vi "Configure Frequency Sweep.vi"(0 "VISA resource name":refnum<visa-resource-name>, 1 "Stop  Frequency (1000 Hz)":dbl=1000.0, 2 "Sweep Hold Time (0 s)":dbl, 5 "Sweep Spacing (0: Linear)":i32(ring) items=["Linear", "Log"], 7 "Sweep Time (1 s)":dbl=1.0, 9 "Channel (1: 1)":i32(ring)=1 items=["1"=1, "2"=2], 11 "error in (no error)":errorcluster, 12 "Start Frequency (100 Hz)":dbl=100.0, 13 "Sweep Return Time (0 s)":dbl) -> (4 "VISA resource name out":refnum<visa-resource-name>, 15 "error out":errorcluster)   [LabVIEW 2019, in "Agilent 3352X Series.lvlib"]
doc: "Configures for a frequency sweep. In the frequency sweep mode, the function generator steps from the start frequency to the stop frequency at a sweep rate. \n\nUse Configure xxx Waveform.VI to change settings for specified waveform before sweeping. You can select a sine, square, ramp, or triangle waveform (pulse, noise, PRBS, arbitrary, and DC are not allowed)."
uses:
  <instrlib>/Agilent 3352X Series/Agilent 3352X Series.lvlib
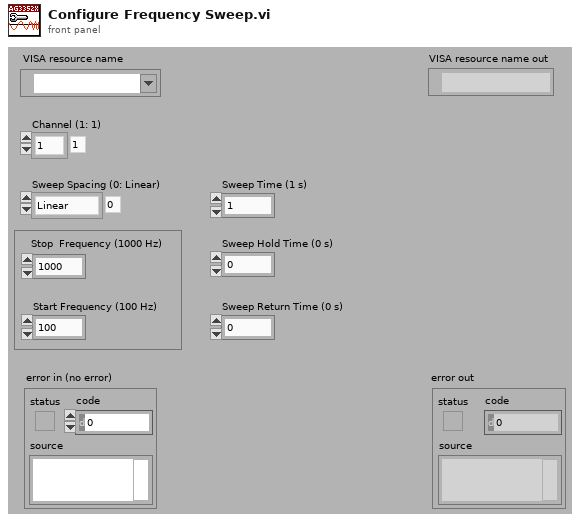
[diagram p1: front panel]
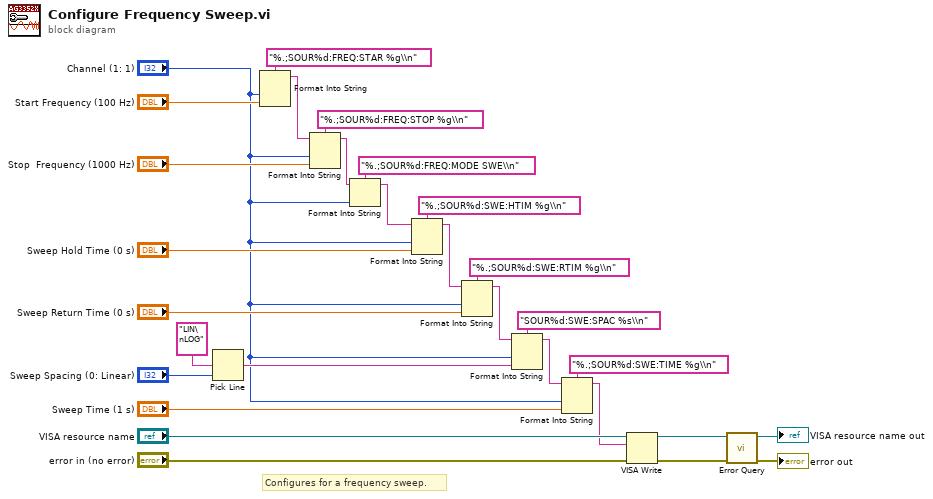
[diagram p0: block diagram]
diagram:
  # "Configures for a frequency sweep."
  n1 = Pick Line(multi-line string="LIN\nLOG", line index="Sweep Spacing (0: Linear)") -> (output string=w20:string)  [unwired: 1 out]
  n2 = Format Into String(format string="%.;SOUR%d:FREQ:STAR %g\\n", "Channel (1: 1)", "Start Frequency (100 Hz)") -> (resulting string=w6:string)  [unwired: 2 in, 1 out]
  n3 = Format Into String(format string="%.;SOUR%d:FREQ:STOP %g\\n", initial string=w6, "Channel (1: 1)", "Stop  Frequency (1000 Hz)") -> (resulting string=w2:string)  [unwired: 1 in, 1 out]
  n4 = Format Into String(format string="%.;SOUR%d:FREQ:MODE SWE\\n", initial string=w2, "Channel (1: 1)") -> (resulting string=w9:string)  [unwired: 1 in, 1 out]
  n5 = Format Into String(format string="%.;SOUR%d:SWE:HTIM %g\\n", initial string=w9, "Channel (1: 1)", "Sweep Hold Time (0 s)") -> (resulting string=w27:string)  [unwired: 1 in, 1 out]
  n6 = Format Into String(format string="%.;SOUR%d:SWE:RTIM %g\\n", initial string=w27, "Channel (1: 1)", "Sweep Return Time (0 s)") -> (resulting string=w22:string)  [unwired: 1 in, 1 out]
  n7 = Format Into String(format string="SOUR%d:SWE:SPAC %s\\n", initial string=w22, "Channel (1: 1)", w20) -> (resulting string=w19:string)  [unwired: 1 in, 1 out]
  n8 = Format Into String(format string="%.;SOUR%d:SWE:TIME %g\\n", initial string=w19, "Channel (1: 1)", "Sweep Time (1 s)") -> (resulting string=w1:string)  [unwired: 1 in, 1 out]
  n9 = VISA Write(VISA resource name="VISA resource name", write buffer=w1, error in (no error)="error in (no error)") -> (VISA resource name out=w13:refnum<visa-resource-name>, error out=w12:errorcluster)  [unwired: 1 out]
  n10 = call <instrlib>:"Error Query.vi"("error in (no error)"=w12, "VISA resource name"=w13) -> ("error out"=→"error out":errorcluster, "VISA resource name out"=→"VISA resource name out":refnum<visa-resource-name>)  [unwired: 8 out]
